vi "TDC_analyseLftFunction.vi"(8 "Error In":errorcluster, 10 "Buffer Size":i32, 11 "Function":u64) -> (0 "Error Out":errorcluster, 1 "Values":dbl[](array[numeric]), 3 "Bin Width":i32, 5 "Size":i32, 7 "Capacity":i32)   [LabVIEW 2011]
uses:
  tdcbase.dll
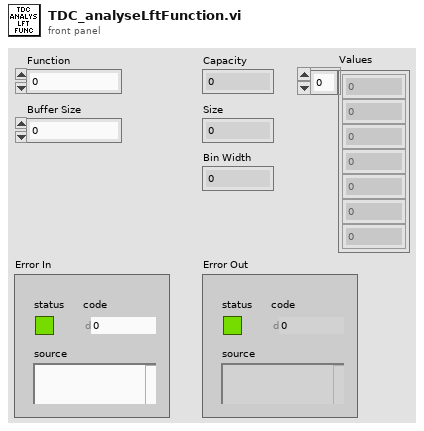
[diagram p1: front panel]
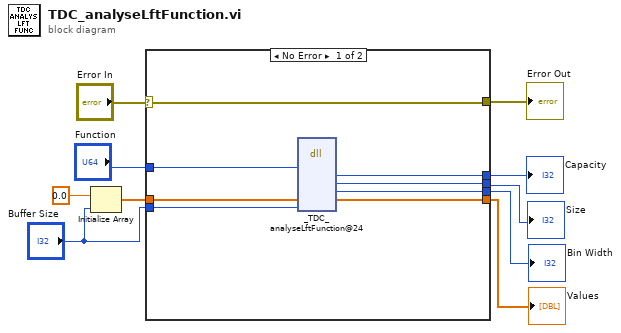
[diagram p0: block diagram]
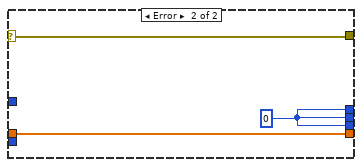
[diagram p2: hidden frame]
diagram:
  n1 = Initialize Array(0.0, "Buffer Size") -> (w6:dbl[])
  n2 = case shown="No Error" "Error In" {
    selector: "Error In" -> [w11 w21]
    tunnel: [w11 w21] -> w9
    tunnel: "Function" -> [w18 _]
    tunnel: w6 -> [w17 w19]
    tunnel: [w16 w19] -> w2
    tunnel: [w15 w20] -> w5
    tunnel: "Buffer Size" -> [w14 _]
    tunnel: [w13 w20] -> w4
    tunnel: [w12 w20] -> w3
    frame No Error {
      n3 = dll-call lib="X:/tdcbase.dll" fn="_TDC_analyseLftFunction@24"("fct"=w18, "values"=w17, "bufSize"=w14) -> ("capacity"=w15:i32, "size"=w13:i32, "binWidth"=w12:i32, "values"=w16:dbl[])  [unwired: 9 in, 2 out]
    }
    frame Error {
      w20 = 0
    }
  }
  "Error Out" <- w9
  "Capacity" <- w5
  "Bin Width" <- w3
  "Size" <- w4
  "Values" <- w2
